vi "Register Callback.vi"(7 "Owner":refnum<class>, 8 "error in (no error)":errorcluster, 9 "Callback":refnum<vi>, 10 "Message ID":string, 11 "Manager in":refnum<class "Manager.lvclass">) -> (0 "error out":errorcluster, 3 "Manager out":refnum<class "Manager.lvclass">)   [LabVIEW 2020, in "Stream-Simple-Msg.lvlib" / "Manager.lvclass"]
uses:
  Manager.lvclass
  Message/Message.lvclass
  Callback.ctl
  Manager.lvclass/Manager.ctl
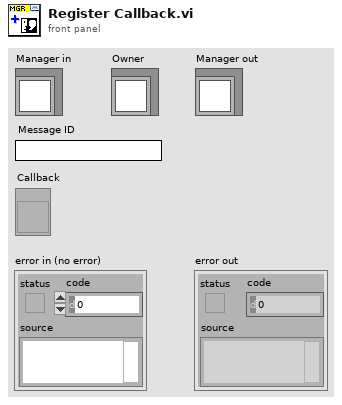
[diagram p1: front panel]
types:
  T1 = typedef "Stream-Simple-Msg.lvlib/Manager.lvclass/Callback.ctl" = cluster{"VI":refnum<vi>, "Owner":refnum<class>}
  T2 = typedef "Stream-Simple-Msg.lvlib/Manager.lvclass/Ref Data.ctl" = cluster{"Message Callbacks":map{string, T1[]}, "Endpoints":map{string, refnum<class "Endpoint.lvclass">}, "Stream Endpoints":refnum<class "Endpoint.lvclass">[], "State Callbacks":T3[]}
  T3 = typedef "Stream-Simple-Msg.lvlib/Manager.lvclass/State Callback.ctl" = cluster{"Owner":refnum<class>, "VI":refnum<vi>}
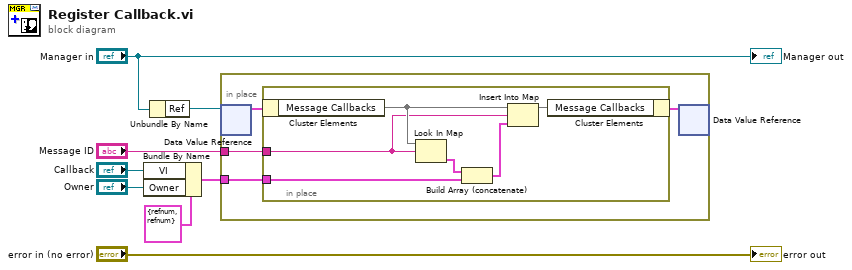
[diagram p0: block diagram]
diagram:
  n1 = Bundle By Name(cluster=T1 {"VI"=refnum, "Owner"=refnum} ("Callback"), "VI"="Callback", "Owner"="Owner") -> (w1:T1)
  n2 = Unbundle By Name("Manager in") -> ("Ref"=w6:refnum<data-value>)
  n3 = in-place {
    in-place-border: "Message ID" -> [w11]
    in-place-border: w1 -> [w10]
    n4 = in-place-dvr #1(w6) -> (w12:T2)  [unwired: 1 out]
    n5 = in-place {
      in-place-border: w11 -> [w15]
      in-place-border: w10 -> [w17]
      n6 = in-place-cluster #2(w12) -> ("Message Callbacks"=w16:map{string, T1[]})
      n7 = Look In Map(map=w16, key=w15) -> (value=w18:T1[])  [unwired: 1 in, 1 out]
      n8 = Build Array (concatenate)(w18, w17) -> (w14:T1[])
      n9 = Insert Into Map(map in=w16, key=w15, value=w14) -> (map out=w13:map{string, T1[]})  [unwired: 2 out]
      n10 = in-place-cluster #2("Message Callbacks"=w13) -> (w9:T2)
    }
    n11 = in-place-dvr #1(w9) -> ()  [unwired: 2 out]
  }
  "error out" <- "error in (no error)"
  "Manager out" <- "Manager in"
